vi "Add Rows.vi"(8 "error in (no error)":errorcluster, 9 "String Data":string[][](array[string]), 11 "DataTable in":refnum<class "DataTable.lvclass">) -> (0 "error out":errorcluster, 3 "DataTable out":refnum<class "DataTable.lvclass">)   [LabVIEW 2014, in "DataGrid.lvlib" / "DataTable.lvclass"]
doc: "This allows any number of rows to be added to the datatable. The data must match the columns defined for the grid."
uses:
  DataTable.lvclass
  DataTable.lvclass/DataTable.ctl
  System.Data
  GridColumn/GridColumn.lvclass/GridColumn.ctl
  GridColumn/Read datatype.vi
  GridColumn/Read Params.vi
  GridColumn/Read Name.vi
  GridColumn/GridColumn.lvclass
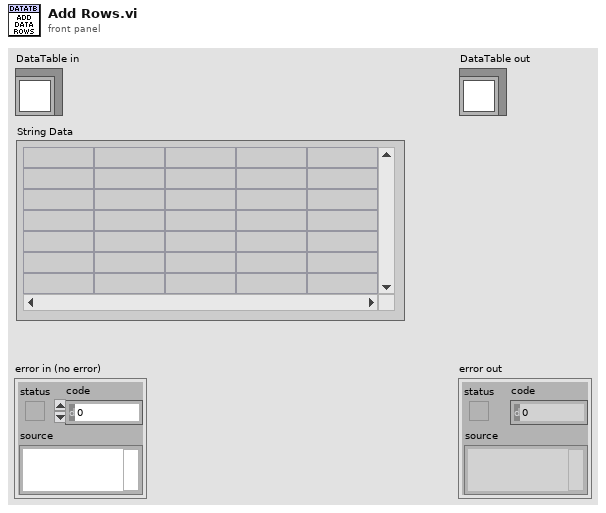
[diagram p1: front panel]
types:
  T1 = typedef "DataGrid.lvlib/GridColumn.lvclass/ColumnType.ctl" = enum16{"string", "image", "check", "numeric", "timestamp", "button", "combo", "link"}
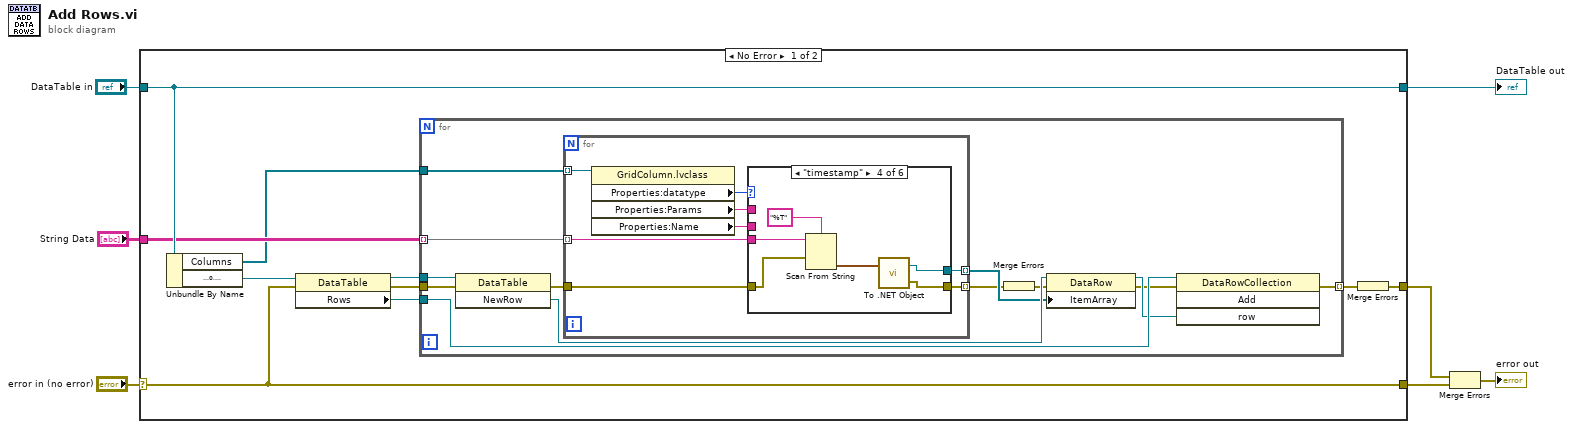
[diagram p0: block diagram]
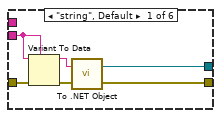
[diagram p2: hidden frame]
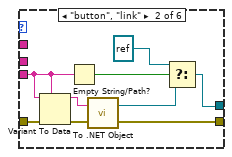
[diagram p3: hidden frame]
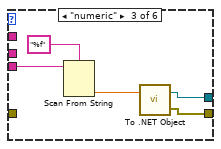
[diagram p4: hidden frame]
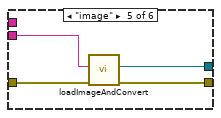
[diagram p5: hidden frame]
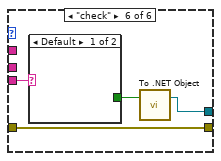
[diagram p6: hidden frame]
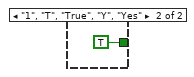
[diagram p7: hidden frame]
diagram:
  n1 = case shown="No Error" "error in (no error)" {
    selector: "error in (no error)" -> [w13 w75]
    tunnel: [w13 w75] -> w6
    tunnel: [w14 w74] -> w4
    tunnel: "DataTable in" -> [w14 w74]
    tunnel: "String Data" -> [w12 _]
    tunnel: [w9 _] -> w1
    frame No Error {
      n2 = Unbundle By Name(w14) -> ("Columns"=w8:refnum<class "GridColumn.lvclass">[], "DataTable"=w11:refnum<k24>)
      n3 = property class="DataTable"(reference=w11, error in=w13) -> (reference out=w10:refnum<k24>, error out=w17:errorcluster, "Rows"=w16:refnum<k24>)
      n4 = for {
        tunnel: w16 -> [w29]
        tunnel: w10 -> [w30]
        tunnel: [w28] -> w15 mode=indexing
        tunnel: w12 -> [w27] mode=indexing
        tunnel: w17 -> [w19]
        tunnel: w8 -> [w18]
        n5 = invoke class="DataTable" method="NewRow"(reference=w30, error in=w19) -> (error out=w26:errorcluster, "NewRow"=w25:refnum<k24>)  [unwired: 1 in, 1 out]
        n6 = for {
          tunnel: w27 -> [w38] mode=indexing
          tunnel: [w37] -> w23 mode=indexing
          tunnel: w26 -> [w36]
          tunnel: [w35] -> w22 mode=indexing
          tunnel: w18 -> [w34] mode=indexing
          n7 = property class="GridColumn.lvclass"(reference=w34) -> ("Properties:datatype"=w33:T1, "Properties:Params"=w32:string, "Properties:Name"=w31:string)  [unwired: 1 in, 2 out]
          n8 = case shown="\"timestamp\"" w33 {
            tunnel: w38 -> [w40 w49 w56 w62 w68 w70]
            tunnel: [w39 w46 w57 w63 w67 w71] -> w37
            tunnel: w36 -> [w43 w52 _ w60 w66 w72]
            tunnel: [w41 w50 w58 w64 w65 w72] -> w35
            tunnel: w32 -> [_ _ _ _ _ _]
            tunnel: w31 -> [_ _ _ _ _ _]
            frame "string", Default {
              n9 = Variant To Data(error in=w43, type=w40, Variant=w40) -> (data=w44:string, error out=w42:errorcluster)
              n10 = call <vilib>:"To .NET Object.vi"("error in (no error)"=w42, "anything"=w44) -> ("error out"=w41:errorcluster, ".NET object"=w39:refnum<k24>)
            }
            frame "button", "link" {
              n11 = Variant To Data(error in=w52, type=w49, Variant=w49) -> (data=w53:string, error out=w51:errorcluster)
              n12 = Empty String/Path?(string/path=w49) -> (empty?=w48:bool)
              n13 = call <vilib>:"To .NET Object.vi"("error in (no error)"=w51, "anything"=w53) -> ("error out"=w50:errorcluster, ".NET object"=w47:refnum<k24>)
              n14 = Select(t=refnum<k24> refnum, s=w48, f=w47) -> (s? t:f=w46:refnum<k24>)
            }
            frame "numeric" {
              n15 = Scan From String(format string="%f", input string=w56) -> (output 1=w54:dbl)  [unwired: 3 in, 3 out]
              n16 = call <vilib>:"To .NET Object.vi"("anything"=w54) -> ("error out"=w58:errorcluster, ".NET object"=w57:refnum<k24>)  [unwired: 1 in]
            }
            frame "timestamp" {
              n17 = Scan From String(format string="%T", input string=w62, error in=w60) -> (output 1=w59:timestamp)  [unwired: 2 in, 3 out]
              n18 = call <vilib>:"To .NET Object.vi"("anything"=w59) -> ("error out"=w64:errorcluster, ".NET object"=w63:refnum<k24>)  [unwired: 1 in]
            }
            frame "image" {
              n19 = call "loadImageAndConvert.vi"("error in (no error)"=w66, "name or relative path"=w68) -> ("error out"=w65:errorcluster, ".NET object"=w67:refnum<k24>)  [unwired: 8 in]
            }
            frame "check" {
              n20 = case shown="Default" w70 {
                tunnel: [_ TRUE] -> w69
                frame Default {
                }
                frame "1", "T", "True", "Y", "Yes" {
                }
              }
              n21 = call <vilib>:"To .NET Object.vi"("anything"=w69) -> (".NET object"=w71:refnum<k24>)  [unwired: 1 in, 1 out]
            }
          }
        }
        n22 = Merge Errors(w22) -> (w21:errorcluster)
        n23 = property class="DataRow"(reference=w25, error in=w21, "ItemArray"=w23) -> (reference out=w24:refnum<k24>, error out=w20:errorcluster)
        n24 = invoke class="DataRowCollection" method="Add"(reference=w29, error in=w20, "row"=w24) -> (error out=w28:errorcluster)  [unwired: 1 in, 3 out]
      }
      n25 = Merge Errors(w15) -> (w9:errorcluster)
    }
    frame Error {
    }
  }
  "DataTable out" <- w4
  n26 = Merge Errors(w1, w6) -> (→"error out":errorcluster)
